vi "Example - Multiple Loggers.vi"() -> ()   [LabVIEW 2020, in "Global_logger.lvlib"]
doc: "Example of logging into UI elements."
uses:
  Global_logger.lvlib
  UI Options.ctl
  General Options.ctl
  Log Fields.ctl
  Level Meaning.ctl
  Sorting.ctl
  New UI Logger.vi
panel:
  in  "Table Control":string[][](table)
  in  "Multicolumn Listbox":i32(listbox)=-1
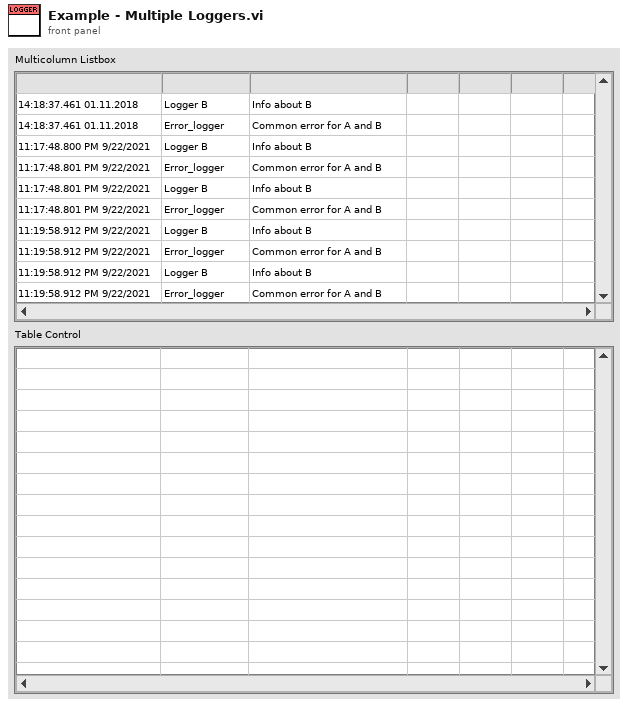
[diagram p1: front panel]
types:
  T1 = typedef "Global_logger.lvlib/General Options.ctl" = cluster{"Format":T2[], "Timestamp format":string, "Level Meaning":T3, "Sorting":T4}
  T2 = typedef "Global_logger.lvlib/Log Fields.ctl" = enum16{"Timestamp", "Level", "Message", "Source VI", "Source App", "Logger Name"}
  T3 = typedef "Global_logger.lvlib/Level Meaning.ctl" = enum16{"Standard", "Positive", "Exact"}
  T4 = typedef "Global_logger.lvlib/Sorting.ctl" = enum16{"Add to Bottom", "Add to Top"}
  T5 = typedef "Global_logger.lvlib/UI Options.ctl" = cluster{"Ctl Refnum":refnum<vi>, "Delimiter":string}
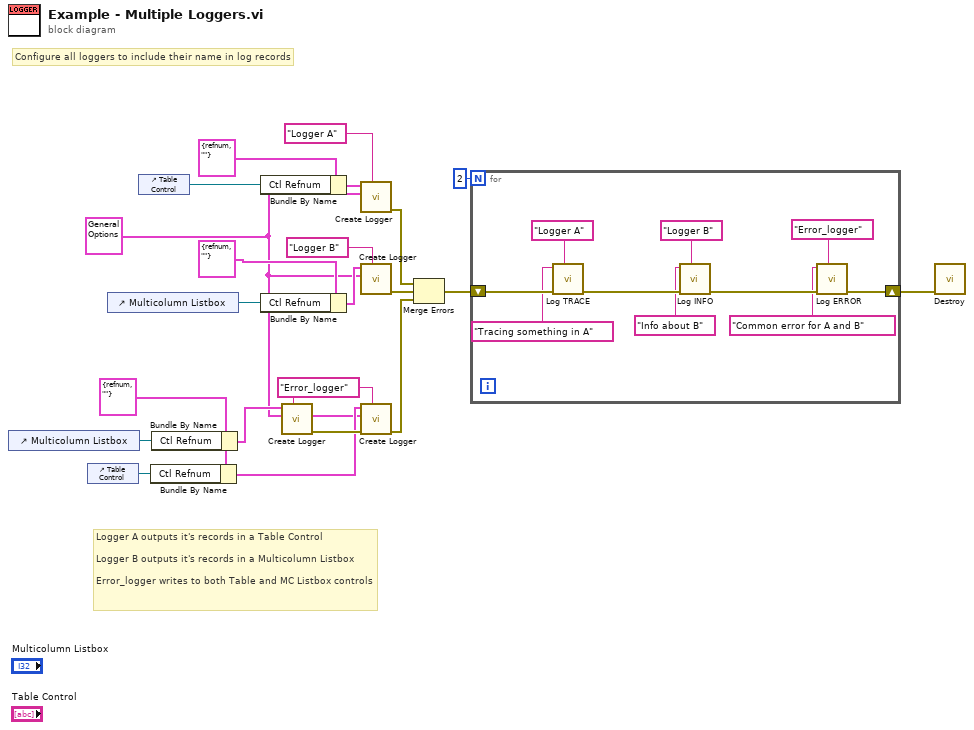
[diagram p0: block diagram]
diagram:
  w3 = T1 {"Format"=[enum."Timestamp", enum."Logger Name", enum."Message"], "Timestamp format"="%T", "Level Meaning"=enum."Standard", "Sorting"=enum."Add to Bottom"} ("General Options")
  w7 = "Error_logger" ("Logger Name")
  w6 = T5 {"Ctl Refnum"=refnum, "Delimiter"=""} ("UI Options")
  # "Logger A outputs it's records in a Table Control\n\nLogger B outputs it's records in a Multicolumn Listbox\n\nError_logger writes to both Table and MC Listbox controls"
  # "Configure all loggers to include their name in log records"
  n1 = control-ref of="Multicolumn Listbox"() -> (w10:refnum<vi>)
  n2 = control-ref of="Table Control"() -> (w4:refnum<vi>)
  n3 = control-ref of="Multicolumn Listbox"() -> (w22:refnum<vi>)
  n4 = control-ref of="Table Control"() -> (w20:refnum<vi>)
  n5 = Bundle By Name(cluster=w6, "Ctl Refnum"=w4) -> (w5:T5)
  n6 = Bundle By Name(cluster=w6, "Ctl Refnum"=w10) -> (w11:T5)
  n7 = Bundle By Name(cluster=T5 {"Ctl Refnum"=refnum, "Delimiter"=""} ("UI Options"), "Ctl Refnum"=w20) -> (w19:T5)
  n8 = Bundle By Name(cluster=T5 {"Ctl Refnum"=refnum, "Delimiter"=""} ("UI Options"), "Ctl Refnum"=w22) -> (w21:T5)
  n9 = call-poly "Create Logger.vi"("Logger Name"=w7, "General Options"=w3, "UI Options"=w11) -> ("error out"=w9:errorcluster)  [unwired: 8 in]
  n10 = call-poly "Create Logger.vi"("Logger Name"="Logger A", "General Options"=w3, "UI Options"=w19) -> ("error out"=w16:errorcluster)  [unwired: 8 in]
  n11 = call-poly "Create Logger.vi"("Logger Name"="Logger B", "General Options"=w3, "UI Options"=w21) -> ("error out"=w15:errorcluster)  [unwired: 8 in]
  n12 = call-poly "Create Logger.vi"("Logger Name"=w7, "error in (no error)"=w9, "General Options"=w3, "UI Options"=w5) -> ("error out"=w8:errorcluster)  [unwired: 7 in]
  n13 = Merge Errors(w16, w15, w8) -> (w12:errorcluster)
  n14 = for {
    N: 2 -> [_]
    shift-right: [w27] -> w1
    shift-left: w12 -> [w32]
    n15 = call "Log TRACE.vi"("Logger Name"="Logger A", "error in (no error)"=w32, "Message"="Tracing something in A") -> ("error out"=w30:errorcluster)  [unwired: 8 in]
    n16 = call "Log INFO.vi"("Logger Name"="Logger B", "error in (no error)"=w30, "Message"="Info about B") -> ("error out"=w28:errorcluster)  [unwired: 8 in]
    n17 = call "Log ERROR.vi"("Logger Name"="Error_logger", "error in (no error)"=w28, "Message"="Common error for A and B") -> ("error out"=w27:errorcluster)  [unwired: 8 in]
  }
  n18 = call "Destroy.vi"("error in (no error)"=w1) -> ()  [unwired: 10 in, 1 out]
